vi "Set Subscription Attribute.vi"(8 "error in (no error)":errorcluster, 10 "Subscription Attribute":T1, 11 "Subscription in":refnum<class "Subscription.lvclass">) -> (0 "error out":errorcluster, 3 "Subscription out":refnum<class "Subscription.lvclass">)   [LabVIEW 2015, in "NI_AWS_SNS.lvlib" / "Subscription.lvclass"]
doc: "Allows a subscription owner to set an attribute of the topic to a new value."
uses:
  Subscription.lvclass
  Subscription Attribute Value Pair.ctl
  Subscription Attribute.ctl
  Core/HTTP Request/Request Options.ctl
  Core/HTTP Request/Name Value Pair.ctl
  Core/HTTP Request/Region handling.ctl
  Core/HTTP Request/URL formatting.ctl
  Core/ARN/ARN.lvclass/ARN.ctl
  Core/ARN/Read ARN.vi
  Core/HTTP Request/HTTP Request.lvclass
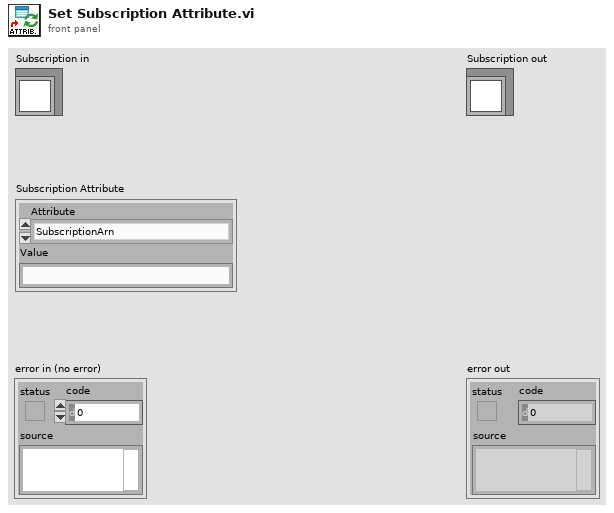
[diagram p1: front panel]
types:
  T1 = typedef "NI_AWS_SNS.lvlib/Subscription.lvclass/Subscription Attribute Value Pair.ctl" = cluster{"Attribute":T2, "Value":string}
  T2 = typedef "NI_AWS_SNS.lvlib/Subscription.lvclass/Subscription Attribute.ctl" = enum16{"SubscriptionArn", "TopicArn", "Owner", "ConfirmationWasAuthenticated", "DeliveryPolicy", "EffectiveDeliveryPolicy", "RawMessageDelivery", "Endpoint", "Protocol"}
  T3 = typedef "NI_AWS_Core.lvlib/HTTP Request.lvclass/Name Value Pair.ctl" = cluster{"name":string, "value":string}
  T4 = typedef "NI_AWS_Core.lvlib/HTTP Request.lvclass/Request Options.ctl" = cluster{"request headers":T3[], "request parameters":T3[], "request body":string, "region handling":T5, "URL formatting":T6}
  T5 = typedef "NI_AWS_Core.lvlib/HTTP Request.lvclass/Region handling.ctl" = enum16{"use region everywhere", "use region (authentication only)", "use region (URL only)", "ignore region everwhere"}
  T6 = typedef "NI_AWS_Core.lvlib/HTTP Request.lvclass/URL formatting.ctl" = enum16{"region-", "region."}
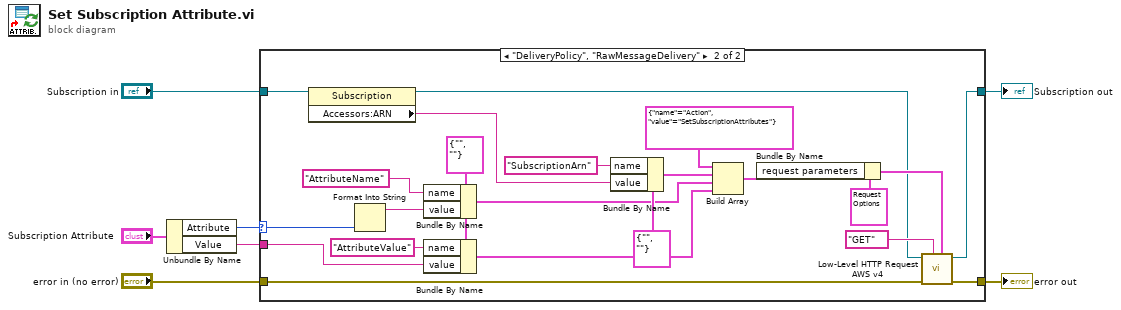
[diagram p0: block diagram]
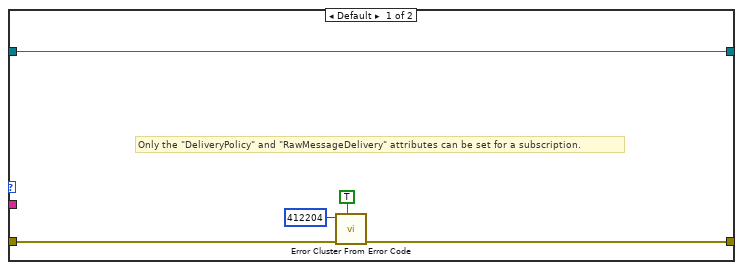
[diagram p2: hidden frame]
diagram:
  n1 = Unbundle By Name("Subscription Attribute") -> ("Attribute"=w2:T2, "Value"=w1:string)
  n2 = case shown="\"DeliveryPolicy\", \"RawMessageDelivery\"" w2 {
    selector: w2 -> [_ w21]
    tunnel: "error in (no error)" -> [w11 w33]
    tunnel: [w10 w32] -> w6
    tunnel: "Subscription in" -> [w12 w31]
    tunnel: [w12 w13] -> w4
    tunnel: w1 -> [_ w19]
    frame Default {
      # "Only the \"DeliveryPolicy\" and \"RawMessageDelivery\" attributes can be set for a subscription."
      n3 = call <vilib>:"Error Cluster From Error Code.vi"("show call chain? (False)"=TRUE, "error in (no error)"=w11, "error code (0)"=412204) -> ("error out"=w10:errorcluster)  [unwired: 6 in]
    }
    frame "DeliveryPolicy", "RawMessageDelivery" {
      w22 = T3 {"name"="", "value"=""} ("element")
      n4 = property class="Subscription"(reference=w31) -> (reference out=w14:refnum<class "Subscription.lvclass">, "Accessors:ARN"=w25:string)  [unwired: 1 in, 1 out]
      n5 = Format Into String(w21) -> (resulting string=w20:string)  [unwired: 3 in, 1 out]
      n6 = Bundle By Name(cluster=w22, "name"="AttributeName", "value"=w20) -> (w24:T3)
      n7 = Bundle By Name(cluster=w22, "name"="AttributeValue", "value"=w19) -> (w23:T3)
      n8 = Bundle By Name(cluster=T3 {"name"="", "value"=""} ("Name Value Pair"), "name"="SubscriptionArn", "value"=w25) -> (w27:T3)
      n9 = Build Array(T3 {"name"="Action", "value"="SetSubscriptionAttributes"} ("Name Value Pair"), w27, w24, w23) -> (w30:T3[])
      n10 = Bundle By Name(cluster=T4 {"request headers"=[], "request parameters"=[], "request body"="", "region handling"=enum."use region everywhere", "URL formatting"=enum."region."} ("Request Options"), "request parameters"=w30) -> (w15:T4)
      n11 = call "Low-Level HTTP Request AWS v4.vi"("Request Options"=w15, "HTTP-Verb"="GET", "error in (no error)"=w33, "AWS Core in"=w14) -> ("error out"=w32:errorcluster, "AWS Core out"=w13:refnum<class "Subscription.lvclass">)  [unwired: 4 in, 2 out]
    }
  }
  "error out" <- w6
  "Subscription out" <- w4
